vi "rt_140_load_boulder_LUT_2.vi"(11 "LUT File":path) -> (1 "Anchor Points":cluster{dbl, dbl}[](array[cluster])=[{-3.141592653589793, 0.0}, {-2.938909256584, 0.03225806451612903}, {-2.736225859578207, 0.06451612903225806}, {-2.533542462572414, 0.0967741935483871}, {-2.330859065566621, 0.12903225806451613}, {-2.1281756685608277, 0.16129032258064516}, {-1.9254922715550344, 0.1935483870967742}, {-1.7228088745492414, 0.22580645161290322}, {-1.5201254775434483, 0.25806451612903225}, {-1.317442080537655, 0.2903225806451613}, {-1.114758683531862, 0.3225806451612903}, {-0.9120752865260688, 0.3548387096774194}, {-0.7093918895202758, 0.3870967741935484}, {-0.5067084925144827, 0.41935483870967744}, {-0.3040250955086896, 0.45161290322580644}, {-0.10134169850289654, 0.4838709677419355}, {0.10134169850289654, 0.5161290322580645}, {0.30402509550868917, 0.5483870967741935}, {0.5067084925144831, 0.5806451612903226}, {0.7093918895202758, 0.6129032258064516}, {0.9120752865260693, 0.6451612903225806}, {1.1147586835318615, 0.6774193548387096}, {1.3174420805376554, 0.7096774193548387}, {1.5201254775434485, 0.7419354838709677}, {1.7228088745492416, 0.7741935483870968}, {1.9254922715550338, 0.8064516129032258}, {2.1281756685608277, 0.8387096774193549}, {2.330859065566621, 0.8709677419354839}, {2.533542462572414, 0.9032258064516129}, {2.736225859578207, 0.9354838709677419}, {2.938909256584, 0.967741935483871}, {3.141592653589793, 1.0}], 2 "'blazing function'":cluster{"X":dbl, "Y":dbl}[](graph)=[{"X"=-3.141592653589793, "Y"=0.0}, {"X"=-2.938909256584, "Y"=0.03225806451612903}, {"X"=-2.736225859578207, "Y"=0.06451612903225806}, {"X"=-2.533542462572414, "Y"=0.0967741935483871}, {"X"=-2.330859065566621, "Y"=0.12903225806451613}, {"X"=-2.1281756685608277, "Y"=0.16129032258064516}, {"X"=-1.9254922715550344, "Y"=0.1935483870967742}, {"X"=-1.7228088745492414, "Y"=0.22580645161290322}, {"X"=-1.5201254775434483, "Y"=0.25806451612903225}, {"X"=-1.317442080537655, "Y"=0.2903225806451613}, {"X"=-1.114758683531862, "Y"=0.3225806451612903}, {"X"=-0.9120752865260688, "Y"=0.3548387096774194}, {"X"=-0.7093918895202758, "Y"=0.3870967741935484}, {"X"=-0.5067084925144827, "Y"=0.41935483870967744}, {"X"=-0.3040250955086896, "Y"=0.45161290322580644}, {"X"=-0.10134169850289654, "Y"=0.4838709677419355}, {"X"=0.10134169850289654, "Y"=0.5161290322580645}, {"X"=0.30402509550868917, "Y"=0.5483870967741935}, {"X"=0.5067084925144831, "Y"=0.5806451612903226}, {"X"=0.7093918895202758, "Y"=0.6129032258064516}, {"X"=0.9120752865260693, "Y"=0.6451612903225806}, {"X"=1.1147586835318615, "Y"=0.6774193548387096}, {"X"=1.3174420805376554, "Y"=0.7096774193548387}, {"X"=1.5201254775434485, "Y"=0.7419354838709677}, {"X"=1.7228088745492416, "Y"=0.7741935483870968}, {"X"=1.9254922715550338, "Y"=0.8064516129032258}, {"X"=2.1281756685608277, "Y"=0.8387096774193549}, {"X"=2.330859065566621, "Y"=0.8709677419354839}, {"X"=2.533542462572414, "Y"=0.9032258064516129}, {"X"=2.736225859578207, "Y"=0.9354838709677419}, {"X"=2.938909256584, "Y"=0.967741935483871}, {"X"=3.141592653589793, "Y"=1.0}], 3 "blazing table":dbl[](array[numeric])=[0.0, 0.03225806451612903, 0.06451612903225806, 0.0967741935483871, 0.12903225806451613, 0.16129032258064516, 0.1935483870967742, 0.22580645161290322, 0.25806451612903225, 0.2903225806451613, 0.3225806451612903, 0.3548387096774194, 0.3870967741935484, 0.41935483870967744, 0.45161290322580644, 0.4838709677419355, 0.5161290322580645, 0.5483870967741935, 0.5806451612903226, 0.6129032258064516, 0.6451612903225806, 0.6774193548387096, 0.7096774193548387, 0.7419354838709677, 0.7741935483870968, 0.8064516129032258, 0.8387096774193549, 0.8709677419354839, 0.9032258064516129, 0.9354838709677419, 0.967741935483871, 1.0])   [LabVIEW 2019]
uses:
  <vilib>/Utility/file.llb/Read From Spreadsheet File (DBL).vi
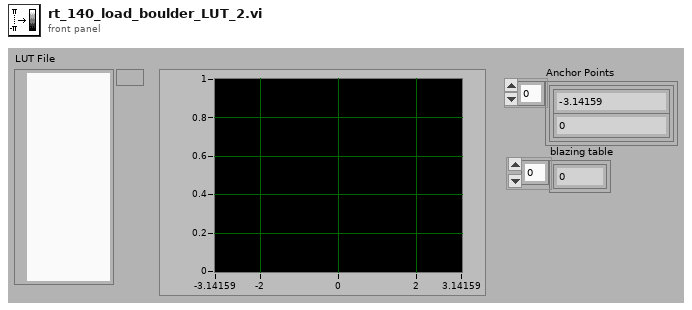
[diagram p1: front panel]
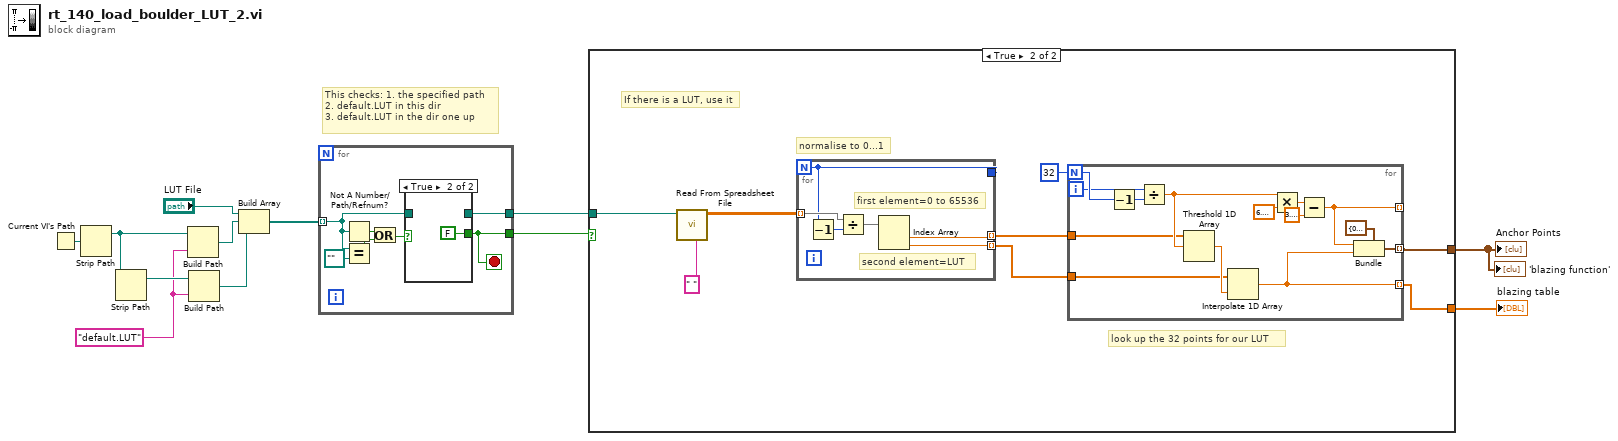
[diagram p0: block diagram]
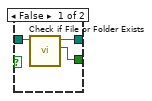
[diagram p2: hidden frame]
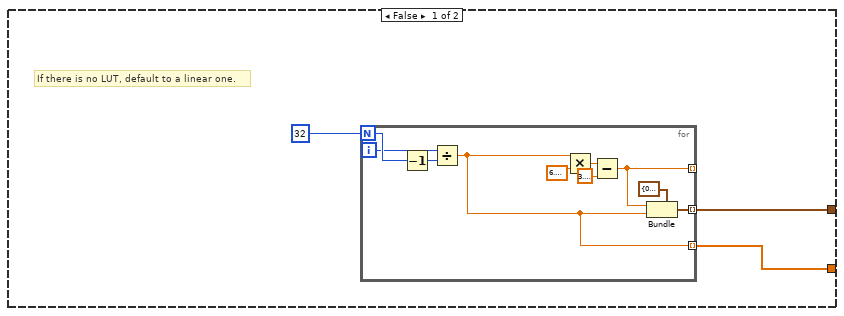
[diagram p3: hidden frame]
diagram:
  w6 = "default.LUT" ("name or relative path")
  # "This checks: 1. the specified path\n2. default.LUT in this dir\n3. default.LUT in the dir one up"
  n1 = Current VI's Path() -> (path=w9:path)
  n2 = Strip Path(path=w9) -> (stripped path=w8:path)  [unwired: 1 out]
  n3 = Strip Path(path=w8) -> (stripped path=w7:path)  [unwired: 1 out]
  n4 = Build Path(base path=w8, name or relative path=w6) -> (appended path=w5:path)
  n5 = Build Path(base path=w7, name or relative path=w6) -> (appended path=w4:path)
  n6 = Build Array("LUT File", w5, w4) -> (w10:path[])
  n7 = for {
    tunnel: w10 -> [w15] mode=indexing
    tunnel: [w18] -> w3
    tunnel: [w13] -> w2
    stop <- w13 stop-if-true
    n8 = Not A Number/Path/Refnum?(number/path/refnum=w15) -> (NaN/Path/Refnum?=w19:bool)
    n9 = Equal?(x=w15, y=path "") -> (x = y?=w16:bool)
    n10 = Or(x=w19, y=w16) -> (x .or. y?=w17:bool)
    n11 = case shown="True" w17 {
      tunnel: w15 -> [w22 _]
      tunnel: [w21 _] -> w18
      tunnel: [w20 FALSE ("file or folder exists?")] -> w13
      frame False {
        n12 = call <vilib>:"Check if File or Folder Exists.vi"("path"=w22) -> ("file or folder exists?"=w20:bool, "dup path"=w21:path)  [unwired: 8 in, 1 out]
      }
      frame True {
      }
    }
  }
  n13 = case shown="True" w2 {
    tunnel: [w25 w39] -> w12
    tunnel: [w26 w38] -> w11
    tunnel: w3 -> [_ w37]
    frame False {
      # "If there is no LUT, default to a linear one."
      n14 = for {
        N: 32 ("Numeric") -> [w32]
        tunnel: [w29] -> _ mode=indexing
        tunnel: [w27] -> w26 mode=indexing
        tunnel: [w28] -> w25 mode=indexing
        i -> [w31]
        n15 = Decrement(x=w32) -> (x-1=w33:i32)
        n16 = Divide(x=w31, y=w33) -> (x/y=w27:dbl)
        n17 = Multiply(x=w27, y=6.283185307179586) -> (x*y=w35:dbl)
        n18 = Subtract(x=w35, y=3.141592653589793) -> (x-y=w29:dbl)
        n19 = Bundle(cluster=cluster{"X":dbl, "Y":dbl} {"X"=0.0, "Y"=0.0} ("Position"), "X"=w29, "Y"=w27) -> (w28:cluster{"X":dbl, "Y":dbl})
      }
    }
    frame True {
      # "If there is a LUT, use it"
      # "look up the 32 points for our LUT"
      # "normalise to 0...1"
      n20 = call-poly <vilib>:"Read From Spreadsheet File.vi"("delimiter (\\t)"=" " ("delimiter (\\t)"), "file path (dialog if empty)"=w37) -> ("all rows"=w43:dbl[][])  [unwired: 5 in, 4 out]
      n21 = for {
        N -> [w62]
        tunnel: w43 -> [w63] mode=indexing
        tunnel: [w62] -> _
        tunnel: [w60] -> w40 mode=indexing
        tunnel: [w59] -> w41 mode=indexing
        # "second element=LUT"
        # "first element=0 to 65536"
        n22 = Decrement(x=w62) -> (x-1=w64:i32)
        n23 = Divide(x=w63, y=w64) -> (x/y=w61:dbl[])
        n24 = Index Array(array=w61) -> (element #1=w59:dbl, element #2=w60:dbl)  [unwired: 2 in]
      }
      n25 = for {
        N: 32 -> [w54]
        tunnel: w41 -> [w51]
        tunnel: [w47] -> _ mode=indexing
        tunnel: w40 -> [w49]
        tunnel: [w46] -> w38 mode=indexing
        tunnel: [w45] -> w39 mode=indexing
        i -> [w53]
        n26 = Decrement(x=w54) -> (x-1=w55:i32)
        n27 = Divide(x=w53, y=w55) -> (x/y=w52:dbl)
        n28 = Threshold 1D Array(2:w52, 3:w51) -> (0:w50:dbl)  [unwired: 1 in]
        n29 = Interpolate 1D Array(1:w50, 2:w49) -> (0:w46:dbl)
        n30 = Multiply(x=w52, y=6.283185307179586) -> (x*y=w57:dbl)
        n31 = Subtract(x=w57, y=3.141592653589793) -> (x-y=w47:dbl)
        n32 = Bundle(cluster=cluster{"X":dbl, "Y":dbl} {"X"=0.0, "Y"=0.0} ("Position"), "X"=w47, "Y"=w46) -> (w45:cluster{"X":dbl, "Y":dbl})
      }
    }
  }
  "'blazing function'" <- w12
  "Anchor Points" <- w12
  "blazing table" <- w11
